vi "Read creates timing source.vi"(8 "error in":errorcluster, 11 "DecideProjectFeatures in":refnum<class "TagBusConfigurablePluginDecideFeatures.lvclass">) -> (0 "error out":errorcluster, 2 "creates timing source":bool, 3 "DecideProjectFeatures out":refnum<class "TagBusConfigurablePluginDecideFeatures.lvclass">)   [LabVIEW 2013, in "TagBusConfigurablePluginDecideFeatures.lvclass"]
uses:
  TagBusConfigurablePluginDecideFeatures.lvclass
  TagBusConfigurablePluginDecideFeatures.lvclass/TagBusConfigurablePluginDecideFeatures.ctl
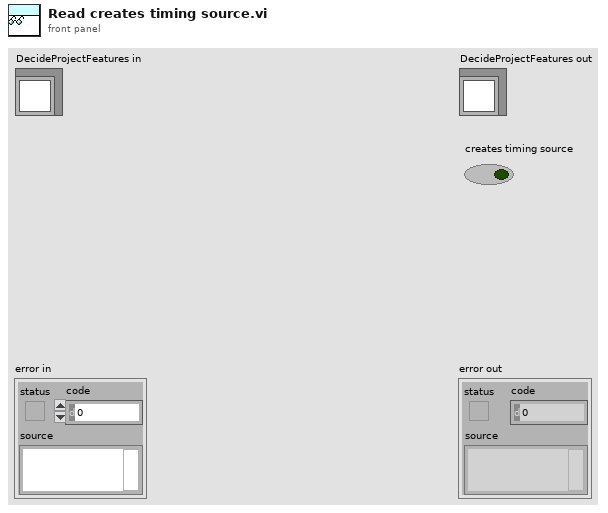
[diagram p1: front panel]
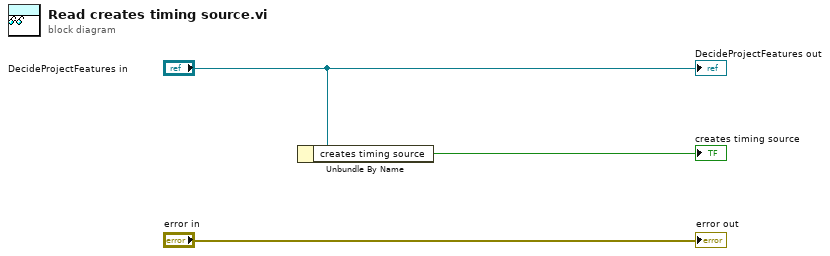
[diagram p0: block diagram]
diagram:
  n1 = Unbundle By Name("DecideProjectFeatures in") -> ("creates timing source"=→"creates timing source":bool)
  "error out" <- "error in"
  "DecideProjectFeatures out" <- "DecideProjectFeatures in"
